vi "Update Tiles.vi"(8 "error in (no error)":errorcluster, 10 "Channel Tiles Info":string[][](array[string]), 11 "Test Channel View in":refnum<class "HVAC System View.lvclass">) -> (0 "error out":errorcluster, 3 "Test Channel View out":refnum<class "HVAC System View.lvclass">)   [LabVIEW 2013, in "HVAC System View.lvlib" / "HVAC System View.lvclass"]
uses:
  HVAC System View.lvclass
  <vilib>/ActorFrameworkMVC/View Actor/View Actor.lvclass/View Actor.ctl
  HVAC System View.lvclass/HVAC System View.ctl
  <vilib>/ActorFrameworkMVC/View Actor/Data Accessors/Get Actor Core VI Reference.vi
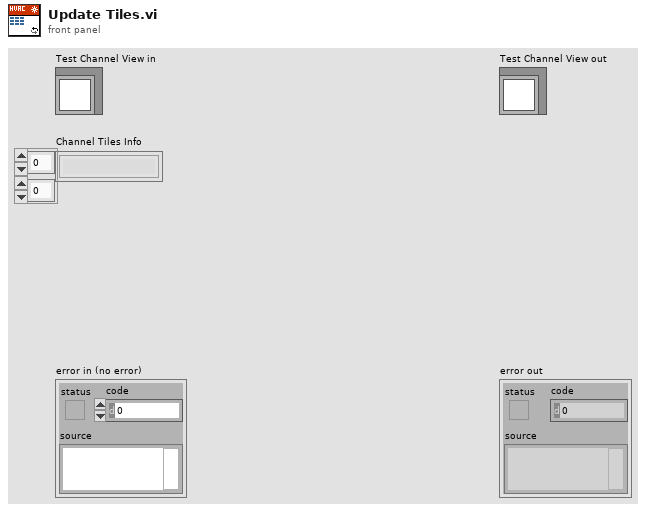
[diagram p1: front panel]
types:
  T1 = cluster{"Channel Tiles Info[0]":string, "Channel Tiles Info[1]":string, "Channel Tiles Info[2]":string}
  T2 = cluster{"[0]":cluster{"Channel Tiles Info[0]":string, "Channel Tiles Info[1]":string, "Channel Tiles Info[2]":string}, "[1]":cluster{"Channel Tiles Info[0]":string, "Channel Tiles Info[1]":string, "Channel Tiles Info[2]":string}, "[2]":cluster{"Channel Tiles Info[0]":string, "Channel Tiles Info[1]":string, "Channel Tiles Info[2]":string}, "[3]":cluster{"Channel Tiles Info[0]":string, "Channel Tiles Info[1]":string, "Channel Tiles Info[2]":string}, "[4]":cluster{"Channel Tiles Info[0]":string, "Channel Tiles Info[1]":string, "Channel Tiles Info[2]":string}, "[5]":cluster{"Channel Tiles Info[0]":string, "Channel Tiles Info[1]":string, "Channel Tiles Info[2]":string}, "[6]":cluster{"Channel Tiles Info[0]":string, "Channel Tiles Info[1]":string, "Channel Tiles Info[2]":string}, "[7]":cluster{"Channel Tiles Info[0]":string, "Channel Tiles Info[1]":string, "Channel Tiles Info[2]":string}, "[8]":cluster{"Channel Tiles Info[0]":string, "Channel Tiles Info[1]":string, "Channel Tiles Info[2]":string}}
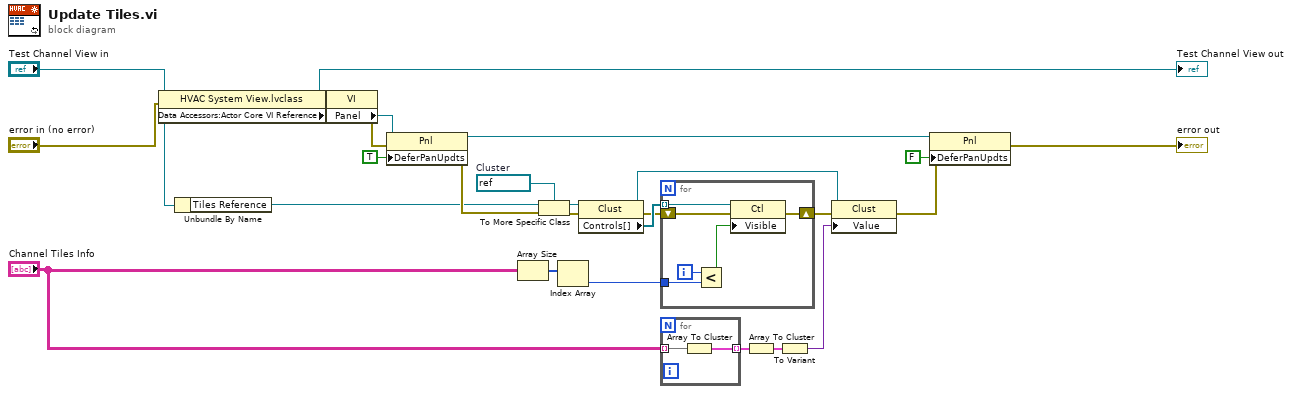
[diagram p0: block diagram]
diagram:
  w19 = refnum<vi> refnum  # Cluster
  n1 = property class="HVAC System View.lvclass"(reference="Test Channel View in", error in="error in (no error)") -> (reference out=→"Test Channel View out":refnum<class "HVAC System View.lvclass">, error out=w3:errorcluster, "Data Accessors:Actor Core VI Reference"=w2:refnum<vi>)
  n2 = Unbundle By Name("Test Channel View in") -> ("Tiles Reference"=w1:refnum<vi>)
  n3 = property class="VI"(reference=w2, error in=w3) -> (error out=w18:errorcluster, "Panel"=w22:refnum<vi>)  [unwired: 1 out]
  n4 = property class="Pnl"(reference=w22, error in=w18, "DeferPanUpdts"=TRUE ("Defer Panel Updates")) -> (reference out=w7:refnum<vi>, error out=w17:errorcluster)
  n5 = Array Size(array="Channel Tiles Info") -> (size(s)=w13:i32[])
  n6 = To More Specific Class(target class=w19, reference=w1, error in=w17) -> (specific class reference=w20:refnum<vi>, error out=w16:errorcluster)
  n7 = Index Array(array=w13) -> (element=w12:i32)  [unwired: 1 in]
  n8 = property on="Property Node" class="Clust"(reference=w20, error in=w16) -> (reference out=w5:refnum<vi>, error out=w14:errorcluster, "Controls[]"=w15:refnum<vi>[])
  n9 = for {
    shift-right: [w33] -> w11
    shift-left: w14 -> [w32]
    tunnel: w15 -> [w31] mode=indexing
    tunnel: w12 -> [w29]
    i -> [w30]
    n10 = Less?(x=w30, y=w29) -> (x < y?=w28:bool)
    n11 = property class="Ctl"(reference=w31, error in=w32, "Visible"=w28) -> (error out=w33:errorcluster)  [unwired: 1 out]
  }
  n12 = for {
    tunnel: "Channel Tiles Info" -> [w35] mode=indexing
    tunnel: [w34] -> w10 mode=indexing
    n13 = Array To Cluster(array=w35) -> (cluster=w34:T1)
  }
  n14 = Array To Cluster(array=w10) -> (cluster=w4:T2)
  n15 = To Variant(anything=w4) -> (Variant=w9:variant)
  n16 = property on="Property Node" class="Clust"(reference=w5, error in=w11, "Value"=w9) -> (error out=w8:errorcluster)  [unwired: 1 out]
  n17 = property class="Pnl"(reference=w7, error in=w8, "DeferPanUpdts"=FALSE ("Defer Panel Updates")) -> (error out=→"error out":errorcluster)  [unwired: 1 out]
